vi "Asylum_SetInWavePair.vi"(4 "decimation":i32, 5 "whichBank":i32, 6 "callback":string, 7 "eventString":string, 8 "error in (no error)":errorcluster, 9 "WaveB":cluster{"channelStringB":string, "waveB":string}, 10 "WaveA":cluster{"channelStringA":string, "waveA":string}, 11 "Application":refnum<k7>) -> (0 "error out":errorcluster, 3 "Application":refnum<k7>)   [LabVIEW 2019]
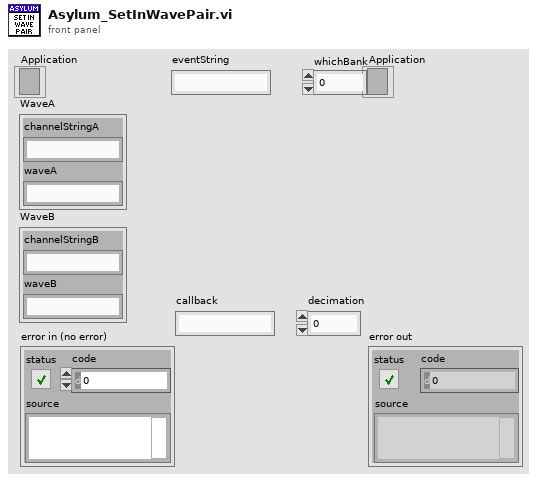
[diagram p1: front panel]
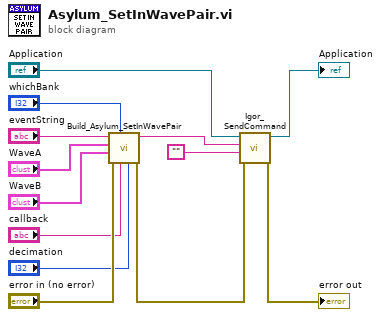
[diagram p0: block diagram]
diagram:
  n1 = call "Build_Asylum_SetInWavePair.vi"("decimation"="decimation", "callback"="callback", "whichBank"="whichBank", "error in (no error)"="error in (no error)", "WaveB"="WaveB", "WaveA"="WaveA", "eventString"="eventString") -> ("error out"=w13:errorcluster, "Command"=w11:string)  [unwired: 3 in]
  n2 = call <userlib>:"Igor_SendCommand.vi"("error in (no error)"=w13, "Format"="", "command"=w11, "Application In"="Application") -> ("error out"=→"error out":errorcluster, "Application Out"=→"Application":refnum<k7>)  [unwired: 4 in, 2 out]
